vi "CTRE_Phoenix_MotorControl_ConfigSlot.vi"(6 "timeoutMs":i32, 7 "Force Write":bool, 8 "error in (no error)":errorcluster, 9 "Slot Number":i32, 10 "Slot Struct":T1, 11 "PhoenixMotorControlDevRef":T2) -> (0 "error out":errorcluster, 3 "PhoenixMotorControlDevRef":T2)   [LabVIEW 2020]
doc: "Sets the slot configurations for the selected slot and motor controller"
uses:
  <vilib>/Rock Robotics/WPI/MotorControl/WPI_MotorControlDeviceRef.ctl
  <vilib>/Rock Robotics/WPI/MotorControl/WPI_MotorControlType.ctl
  <vilib>/Rock Robotics/SystemInterfaces/DIO/FPGA_DIOPWMChannel.ctl
  <vilib>/Rock Robotics/WPI/PWM/WPI_PWMDeadband.ctl
  <vilib>/Rock Robotics/SystemInterfaces/DIO/FPGA_DIOChannel.ctl
  <vilib>/Rock Robotics/WPI/ThirdParty/Phoenix-LabVIEW/Motor Controller/Controls/CTRE_Phoenix_MotorControl_SlotStructure.ctl
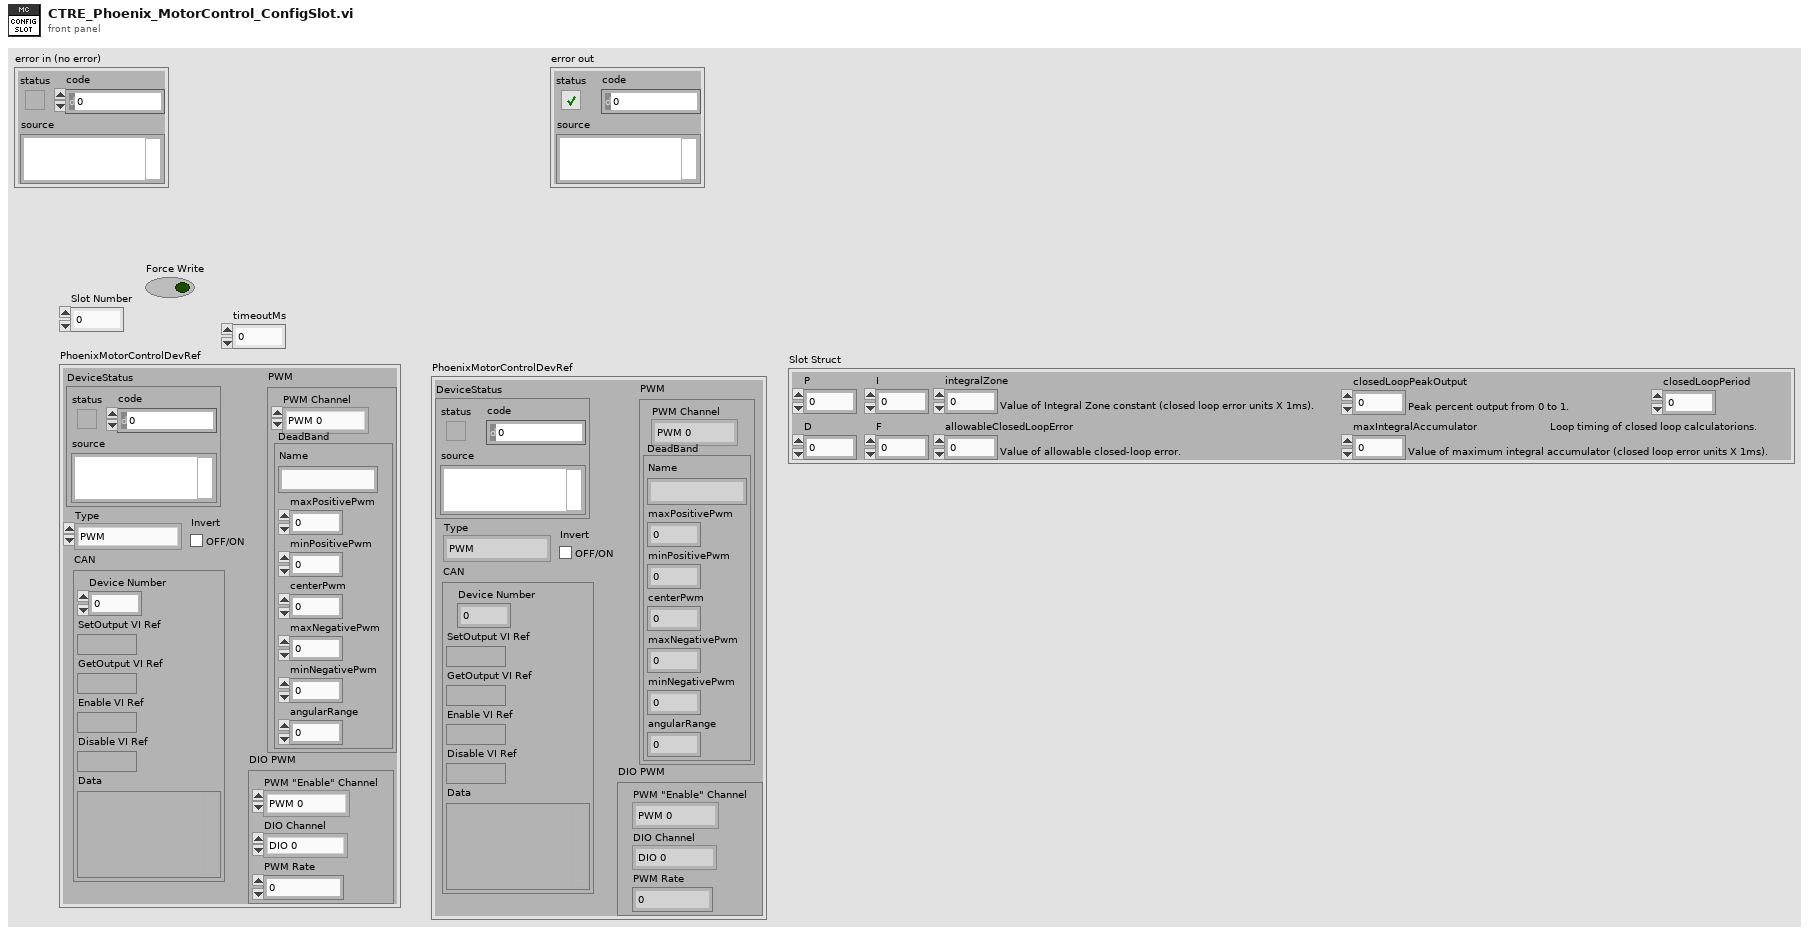
[diagram p1: front panel]
types:
  T1 = typedef "CTRE_Phoenix_MotorControl_SlotStructure.ctl" = cluster{"P":dbl, "I":dbl, "D":dbl, "F":dbl, "integralZone":dbl, "allowableClosedLoopError":i32, "maxIntegralAccumulator":dbl, "closedLoopPeakOutput":dbl, "closedLoopPeriod":i32}
  T2 = typedef "WPI_MotorControlDeviceRef.ctl" = cluster{"DeviceStatus":errorcluster, "Type":T3, "PWM":cluster{"PWM Channel":T4, "DeadBand":T5}, "CAN":cluster{"Device Number":u8, "SetOutput VI Ref":variant, "GetOutput VI Ref":variant, "Enable VI Ref":variant, "Disable VI Ref":variant, "Data":variant}, "Invert":bool, "DIO PWM":cluster{"PWM \"Enable\" Channel":T4, "DIOChannel":T6, "PWM Rate":dbl}}
  T3 = typedef "WPI_MotorControlType.ctl" = enum16{"PWM", "CAN", "DIO PWM"}
  T4 = typedef "FPGA_DIOPWMChannel.ctl" = enum8{"PWM 0", "PWM 1", "PWM 2", "PWM 3", "PWM 4", "PWM 5", "PWM 6", "PWM 7", "PWM 8", "PWM 9", "PWM MXP 0", "PWM MXP 1", "PWM MXP 2", "PWM MXP 3", "PWM MXP 4", "PWM MXP 5", "PWM MXP 6", "PWM MXP 7", "PWM MXP 8", "PWM MXP 9", "Invalid"}
  T5 = typedef "WPI_PWMDeadband.ctl" = cluster{"Name":string, "maxPositivePwm":i32, "minPositivePwm":i32, "centerPwm":i32, "maxNegativePwm":i32, "minNegativePwm":i32, "angularRange":u16}
  T6 = typedef "FPGA_DIOChannel.ctl" = enum8{"DIO 0", "DIO 1", "DIO 2", "DIO 3", "DIO 4", "DIO 5", "DIO 6", "DIO 7", "DIO 8", "DIO 9", "DIO MXP 0", "DIO MXP 1", "DIO MXP 2", "DIO MXP 3", "DIO MXP 4", "DIO MXP 5", "DIO MXP 6", "DIO MXP 7", "DIO MXP 8", "DIO MXP 9", "DIO MXP 10", "DIO MXP 11", "DIO MXP 12", "DIO MXP 13", "DIO MXP 14", "DIO MXP 15", "SPI Port CS1", "SPI Port CS2", "SPI Port CS3", "SPI Port MISO", "SPI Port MOSI", "Invalid"}
  T7 = cluster{"P":bool, "I":bool, "D":bool, "F":bool, "integralZone":bool, "allowableClosedLoopError":bool, "maxIntegralAccumulator":bool, "closedLoopPeakOutput":bool, "closedLoopPeriod":bool}
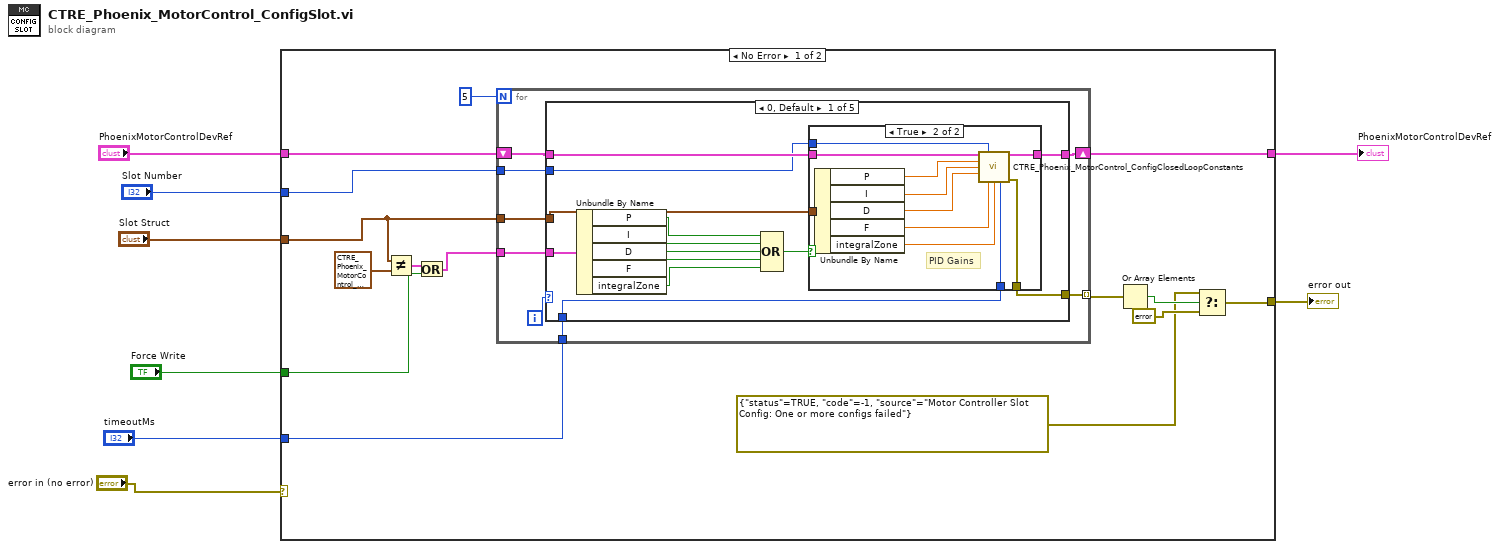
[diagram p0: block diagram]
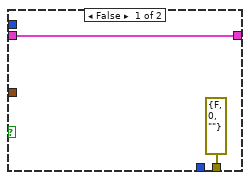
[diagram p2: hidden frame]
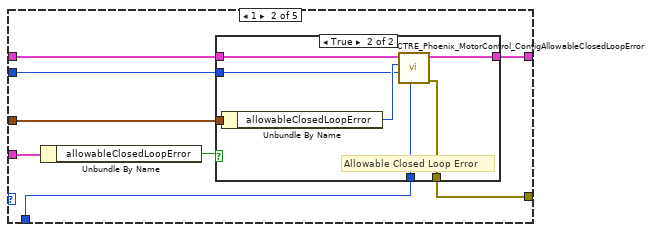
[diagram p3: hidden frame]
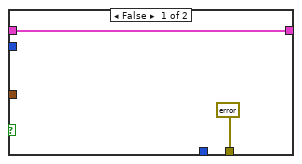
[diagram p4: hidden frame]
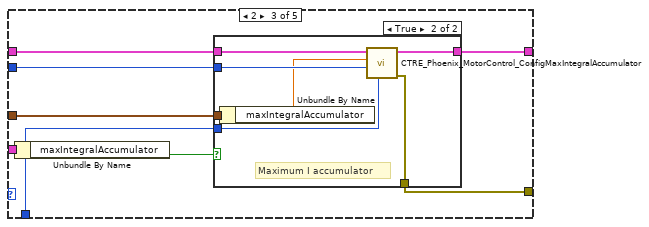
[diagram p5: hidden frame]
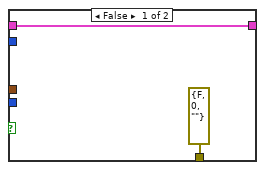
[diagram p6: hidden frame]
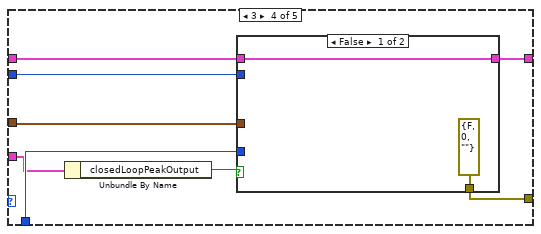
[diagram p7: hidden frame]
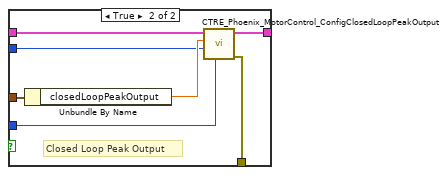
[diagram p8: hidden frame]
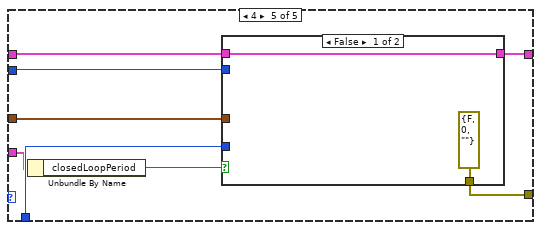
[diagram p9: hidden frame]
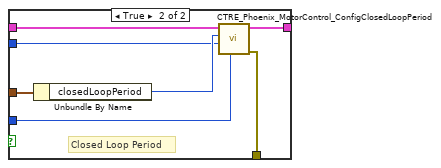
[diagram p10: hidden frame]
diagram:
  n1 = case shown="No Error" "error in (no error)" {
    selector: "error in (no error)" -> [_ w127]
    tunnel: "timeoutMs" -> [w22 _]
    tunnel: "Slot Number" -> [w21 _]
    tunnel: [w20 w126] -> w6
    tunnel: "PhoenixMotorControlDevRef" -> [w19 w126]
    tunnel: "Slot Struct" -> [w17 _]
    tunnel: "Force Write" -> [w15 _]
    tunnel: [w10 w127] -> w2
    frame No Error {
      n2 = Not Equal?(x=w17, y=T1 {"P"=0.0, "I"=0.0, "D"=0.0, "F"=0.0, "integralZone"=0.0, "allowableClosedLoopError"=0, "maxIntegralAccumulator"=0.0, "closedLoopPeakOutput"=1.0, "closedLoopPeriod"=1}) -> (x != y?=w14:T7)
      n3 = Or(x=w14, y=w15) -> (x .or. y?=w13:T7)
      n4 = for {
        N: 5 -> [_]
        tunnel: w17 -> [w30]
        shift-right: [w28] -> w20
        shift-left: w19 -> [w29]
        tunnel: [w27] -> w18 mode=indexing
        tunnel: w21 -> [w26]
        tunnel: w22 -> [w25]
        tunnel: w13 -> [w24]
        i -> [w31]
        n5 = case shown="0, Default" w31 {
          tunnel: w30 -> [w44 w65 w82 w99 w116]
          tunnel: w29 -> [w43 w64 w81 w97 w114]
          tunnel: [w42 w63 w80 w98 w115] -> w28
          tunnel: [w41 w61 w77 w94 w111] -> w27
          tunnel: w26 -> [w40 w62 w79 w96 w113]
          tunnel: w25 -> [w39 w60 w78 w95 w112]
          tunnel: w24 -> [w38 w59 w76 w93 w110]
          frame 0, Default {
            n6 = Unbundle By Name(w38) -> ("P"=w37:bool, "I"=w36:bool, "D"=w35:bool, "F"=w34:bool, "integralZone"=w33:bool)
            n7 = Compound Arithmetic op=OR(w37, w36, w35, w34, w33) -> (w32:bool)
            n8 = case shown="True" w32 {
              tunnel: w44 -> [_ w57]
              tunnel: w43 -> [w46 w56]
              tunnel: [w46 w55] -> w42
              tunnel: [errorcluster {"status"=FALSE, "code"=0, "source"=""} ("error out") w54] -> w41
              tunnel: w40 -> [_ w48]
              tunnel: w39 -> [_ w47]
              frame False {
              }
              frame True {
                # "PID Gains"
                n9 = Unbundle By Name(w57) -> ("P"=w53:dbl, "I"=w52:dbl, "D"=w51:dbl, "F"=w50:dbl, "integralZone"=w49:dbl)
                n10 = call <vilib>:"CTRE_Phoenix_MotorControl_ConfigClosedLoopConstants.vi"("PhoenixMotorControlDevRef"=w56, "slotIdx"=w48, "P"=w53, "I"=w52, "D"=w51, "F"=w50, "I Zone"=w49, "timeoutMs"=w47) -> ("PhoenixMotorControlDevRef"=w55:T2, "error out"=w54:errorcluster)  [unwired: 6 in]
              }
            }
          }
          frame 1 {
            n11 = Unbundle By Name(w59) -> ("allowableClosedLoopError"=w58:bool)
            n12 = case shown="True" w58 {
              tunnel: w65 -> [_ w74]
              tunnel: w64 -> [w67 w73]
              tunnel: [w67 w72] -> w63
              tunnel: w62 -> [_ w70]
              tunnel: [errorcluster {"status"=FALSE, "code"=0, "source"=""} ("error out") w69] -> w61
              tunnel: w60 -> [_ w68]
              frame False {
              }
              frame True {
                # "Allowable Closed Loop Error"
                n13 = Unbundle By Name(w74) -> ("allowableClosedLoopError"=w71:i32)
                n14 = call <vilib>:"CTRE_Phoenix_MotorControl_ConfigAllowableClosedLoopError.vi"("timeoutMs"=w68, "slotIdx"=w70, "allowableClosedLoopError"=w71, "PhoenixMotorControlDevRef"=w73) -> ("error out"=w69:errorcluster, "PhoenixMotorControlDevRef"=w72:T2)  [unwired: 6 in]
              }
            }
          }
          frame 2 {
            n15 = Unbundle By Name(w76) -> ("maxIntegralAccumulator"=w75:bool)
            n16 = case shown="True" w75 {
              tunnel: w82 -> [_ w91]
              tunnel: w81 -> [w84 w90]
              tunnel: [w84 w89] -> w80
              tunnel: w79 -> [_ w88]
              tunnel: w78 -> [_ w86]
              tunnel: [errorcluster {"status"=FALSE, "code"=0, "source"=""} ("error out") w85] -> w77
              frame False {
              }
              frame True {
                # "Maximum I accumulator"
                n17 = Unbundle By Name(w91) -> ("maxIntegralAccumulator"=w87:dbl)
                n18 = call <vilib>:"CTRE_Phoenix_MotorControl_ConfigMaxIntegralAccumulator.vi"("timeoutMs"=w86, "slotIdx"=w88, "Maximum Integral Accumulator Value"=w87, "PhoenixMotorControlDevRef"=w90) -> ("error out"=w85:errorcluster, "PhoenixMotorControlDevRef"=w89:T2)  [unwired: 6 in]
              }
            }
          }
          frame 3 {
            n19 = Unbundle By Name(w93) -> ("closedLoopPeakOutput"=w92:bool)
            n20 = case shown="False" w92 {
              tunnel: w99 -> [_ w108]
              tunnel: [w101 w107] -> w98
              tunnel: w97 -> [w101 w106]
              tunnel: w96 -> [_ w104]
              tunnel: w95 -> [_ w103]
              tunnel: [errorcluster {"status"=FALSE, "code"=0, "source"=""} ("error out") w102] -> w94
              frame False {
              }
              frame True {
                # "Closed Loop Peak Output"
                n21 = Unbundle By Name(w108) -> ("closedLoopPeakOutput"=w105:dbl)
                n22 = call <vilib>:"CTRE_Phoenix_MotorControl_ConfigClosedLoopPeakOutput.vi"("timoutMs"=w103, "slotIdx"=w104, "peakOutput"=w105, "PhoenixMotorControlDevRef"=w106) -> ("error out"=w102:errorcluster, "PhoenixMotorControlDevRef"=w107:T2)  [unwired: 6 in]
              }
            }
          }
          frame 4 {
            n23 = Unbundle By Name(w110) -> ("closedLoopPeriod"=w109:bool)
            n24 = case shown="False" w109 {
              tunnel: w116 -> [_ w125]
              tunnel: [w118 w124] -> w115
              tunnel: w114 -> [w118 w123]
              tunnel: w113 -> [_ w121]
              tunnel: w112 -> [_ w120]
              tunnel: [errorcluster {"status"=FALSE, "code"=0, "source"=""} ("error out") w119] -> w111
              frame False {
              }
              frame True {
                # "Closed Loop Period"
                n25 = Unbundle By Name(w125) -> ("closedLoopPeriod"=w122:i32)
                n26 = call <vilib>:"CTRE_Phoenix_MotorControl_ConfigClosedLoopPeriod.vi"("timoutMs"=w120, "slotIdx"=w121, "loopTimeMs"=w122, "PhoenixMotorControlDevRef"=w123) -> ("error out"=w119:errorcluster, "PhoenixMotorControlDevRef"=w124:T2)  [unwired: 6 in]
              }
            }
          }
        }
      }
      n27 = Or Array Elements(Boolean array=w18) -> (logical OR=w12:bool)
      n28 = Select(t=errorcluster {"status"=TRUE, "code"=-1, "source"="Motor Controller Slot Config: One or more configs failed"}, s=w12, f=errorcluster {"status"=FALSE, "code"=0, "source"=""} ("error out")) -> (s? t:f=w10:errorcluster)
    }
    frame Error {
    }
  }
  "PhoenixMotorControlDevRef" <- w6
  "error out" <- w2
